vi "1BS3HD_Convert_HD_v00.vi"(8 "Extras Homodyne":T1, 11 "PII Control":T2={"P Gain"=0, "P Bit Shift"=1, "I Bit Shift"=0, "I Gain"=1, "Lock Threshold"=20, "Lock"=FALSE, "Hold"=FALSE, "Scan Frequency"=65509, "Scan Bit Shift"=20, "Gains +/- "=FALSE, "Pre- Offset x"=-5.0, "Pre-Offset p"=8.0, "Gain Error x"=-5, "Lock Angle"=0.0, "Gain Error p\n\n"=-4} {"Lock Angle" min=-90.0 max=90.0 scale=-90.0..90.0 scale format="%#_2g"; "Pre-Offset p" scale=-0.01..0.01 scale format="%#_5f"; "Pre- Offset x" scale=-0.01..0.01 scale format="%#_5f"; "Scan Frequency" scale=1.0..30.0; "I Gain" scale=0.0..50.0; "P Gain" scale=0.0..50.0}) -> (3 "PII+Error":T11)   [LabVIEW 2013]
uses:
  Strict Type Defs/PII individual.ctl
  Strict Type Defs/Errors Converted Graph HD.ctl
  Strict Type Defs/PII and Error Graph HD.ctl
  Strict Type Defs/1BS3HD Control GUI HD.ctl
  Strict Type Defs/PII Gains.ctl
  Strict Type Defs/I16 white control.ctl
  Strict Type Defs/Thresh slider.ctl
  Strict Type Defs/Lock or Hold.ctl
  Strict Type Defs/Scan Freq Slider.ctl
  Strict Type Defs/Gains negative horizontal.ctl
  Strict Type Defs/Slider and display.ctl
  Strict Type Defs/theta 1SDI.ctl
  Strict Type Defs/Extras PII 1SDI HD.ctl
panel:
  in  "PII+Error type def":T11
  in  "Error individual":T12
  in  "PII In typdef":T13
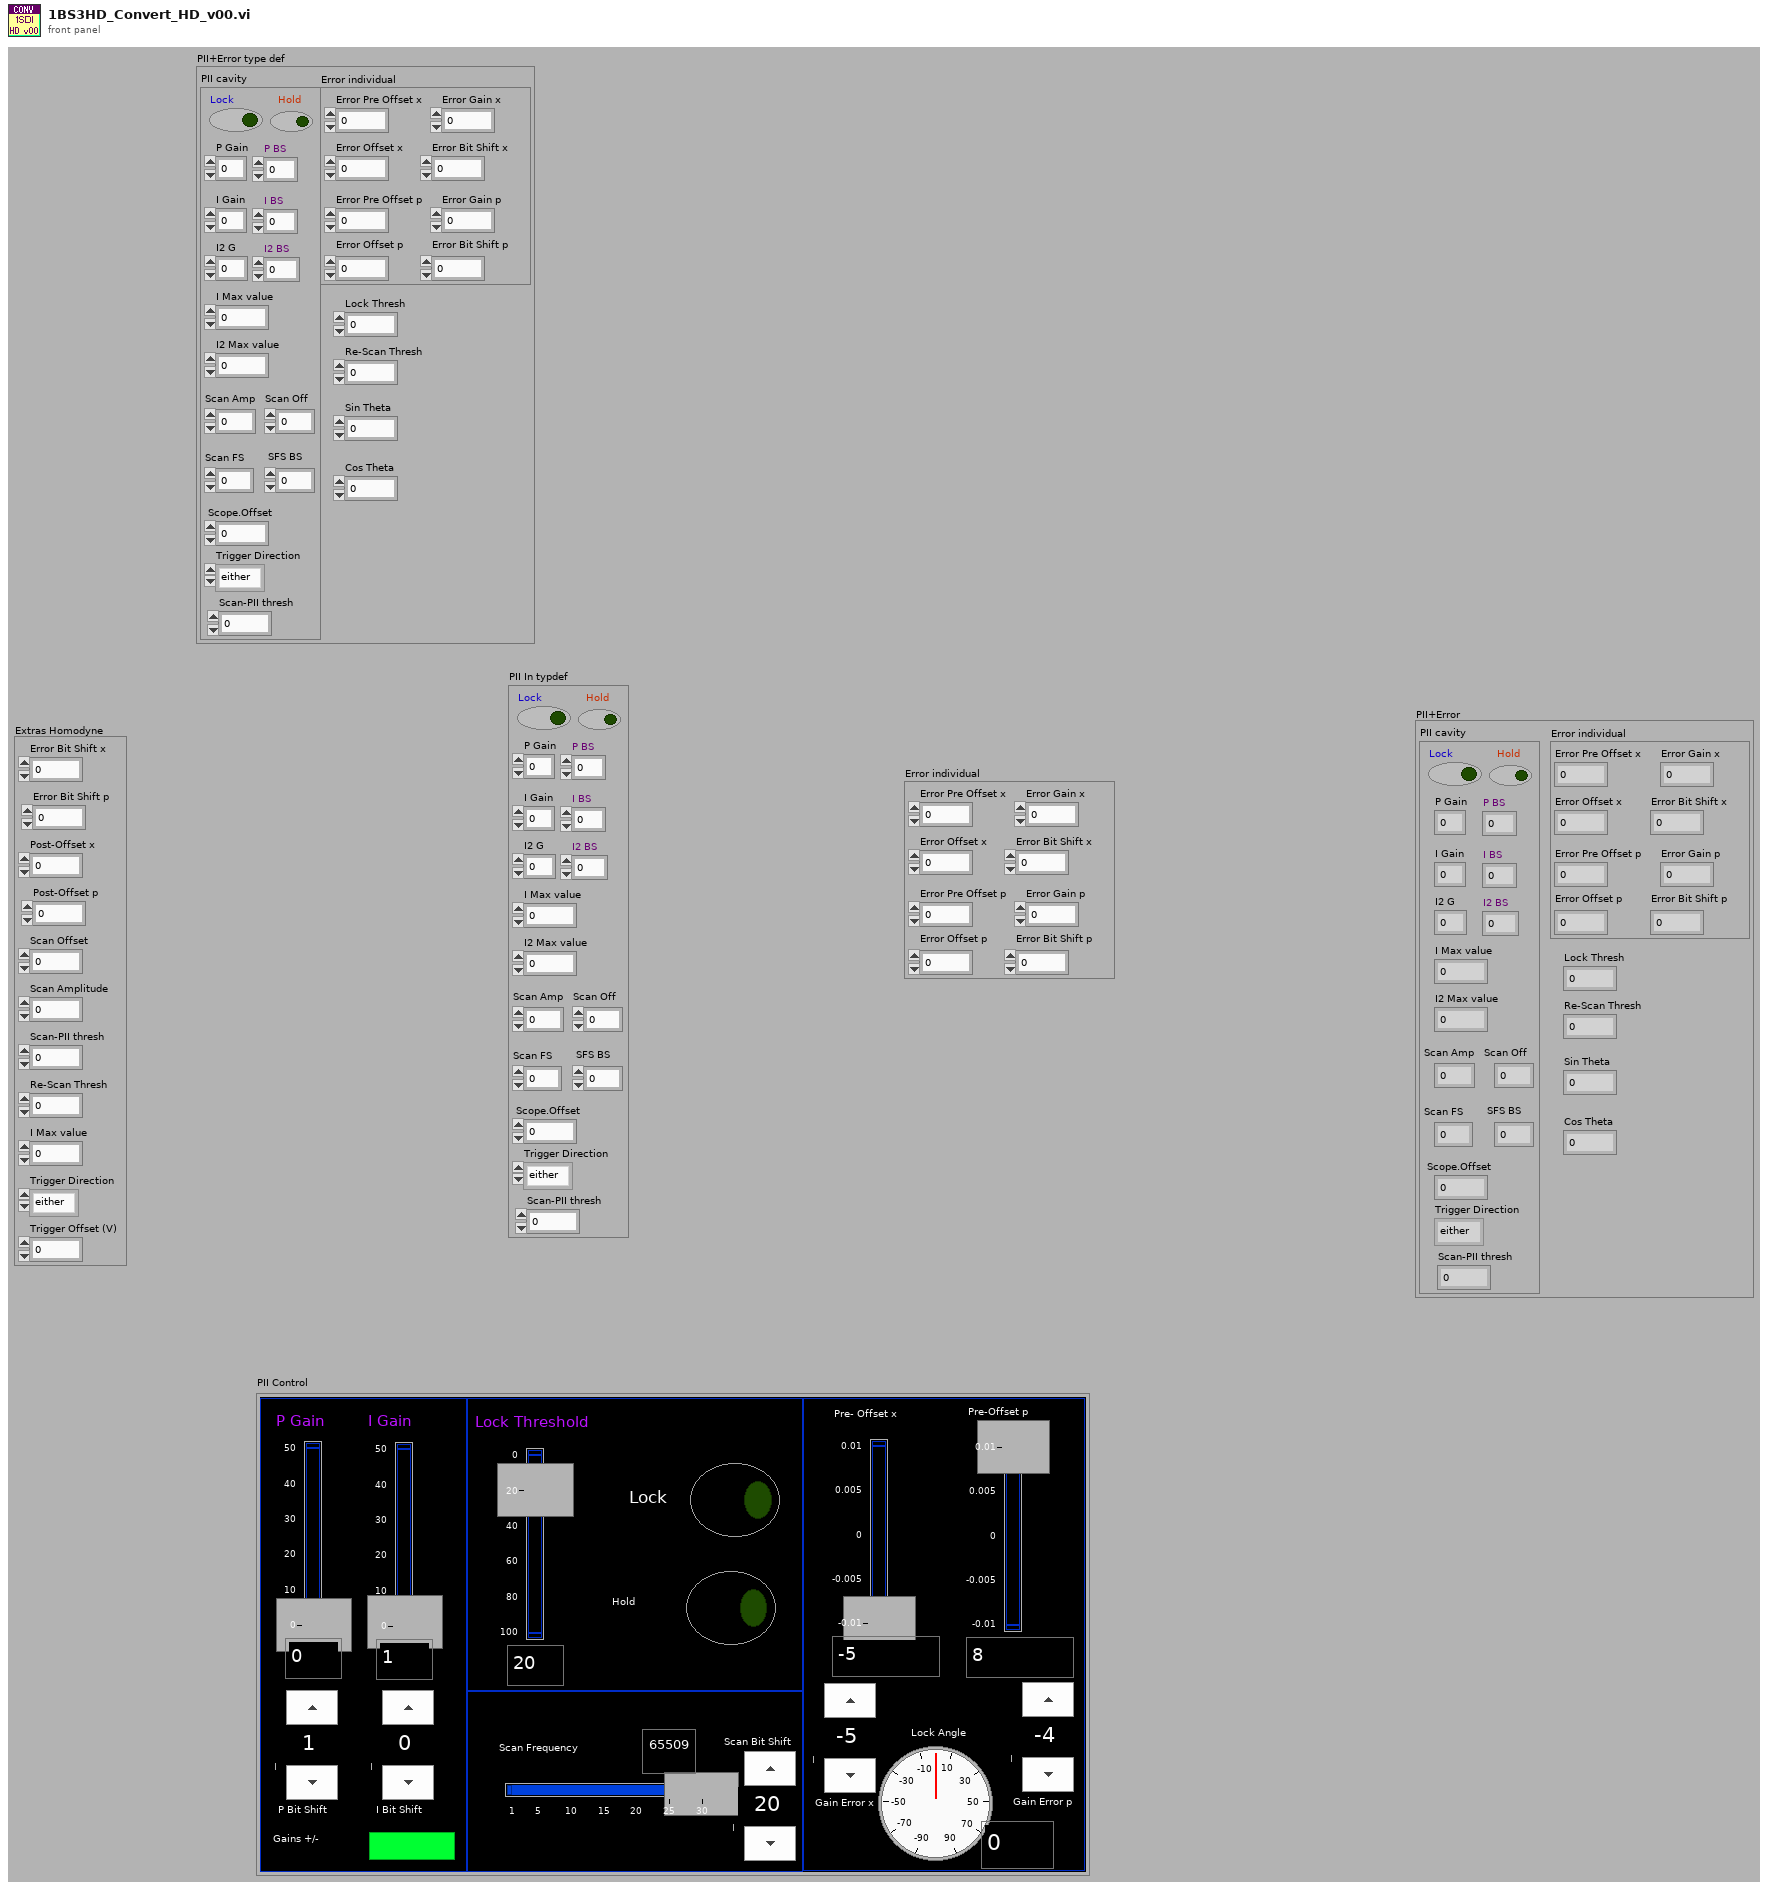
[diagram p1: front panel]
types:
  T1 = typedef "Extras PII 1SDI HD.ctl" = cluster{"Error Bit Shift p":i16, "Scan Offset":dbl, "Scan Amplitude":dbl, "Scan-PII thresh":i16, "Re-Scan Thresh":i16, "I Max value":i32, "Trigger Direction":enum8{"either", "minus-plus", "plus-minus"}, "Trigger Offset (V)":dbl, "Error Bit Shift x":i16, "Post-Offset p":dbl, "Post-Offset x":dbl}
  T2 = typedef "1BS3HD Control GUI HD.ctl" = cluster{"P Gain":T3, "P Bit Shift":T4, "I Bit Shift":T4, "I Gain":T3, "Lock Threshold":T5, "Lock":T6, "Hold":T6, "Scan Frequency":T7, "Scan Bit Shift":T4, "Gains +/- ":T8, "Pre- Offset x":T9, "Pre-Offset p":T9, "Gain Error x":T4, "Lock Angle":T10, "Gain Error p\n\n":T4}
  T3 = typedef "PII Gains.ctl" = i32
  T4 = typedef "I16 white control.ctl" = i16
  T5 = typedef "Thresh slider.ctl" = i16
  T6 = typedef "Lock or Hold.ctl" = bool
  T7 = typedef "Scan Freq Slider.ctl" = u16
  T8 = typedef "Gains negative horizontal.ctl" = bool
  T9 = typedef "Slider and display.ctl" = dbl
  T10 = typedef "theta 1SDI.ctl" = dbl
  T11 = typedef "PII and Error Graph HD.ctl" = cluster{"Error individual":T12, "PII cavity":T13, "Lock Thresh":i16, "Re-Scan Thresh":i16, "Sin Theta":i32, "Cos Theta":i32}
  T12 = typedef "Errors Converted Graph HD.ctl" = cluster{"Error Pre Offset x":i16, "Error Offset x":i16, "Error Gain x":i16, "Error Bit Shift x":i16, "Error Pre Offset p":i16, "Error Offset p":i16, "Error Gain p":i16, "Error Bit Shift p":i16}
  T13 = typedef "PII individual.ctl" = cluster{"Lock":bool, "Hold":bool, "P Gain":i32, "P BS":i16, "I Gain":i32, "I BS":i16, "I2 G":i32, "I2 BS":i16, "Scan Amp":i16, "Scan Off":i16, "Scan FS":u16, "SFS BS":i16, "I Max value":i32, "I2 Max value":i32, "Scope.Offset":i16, "Trigger Direction":enum8{"either", "minus-plus", "plus-minus"}, "Scan-PII thresh":i16}
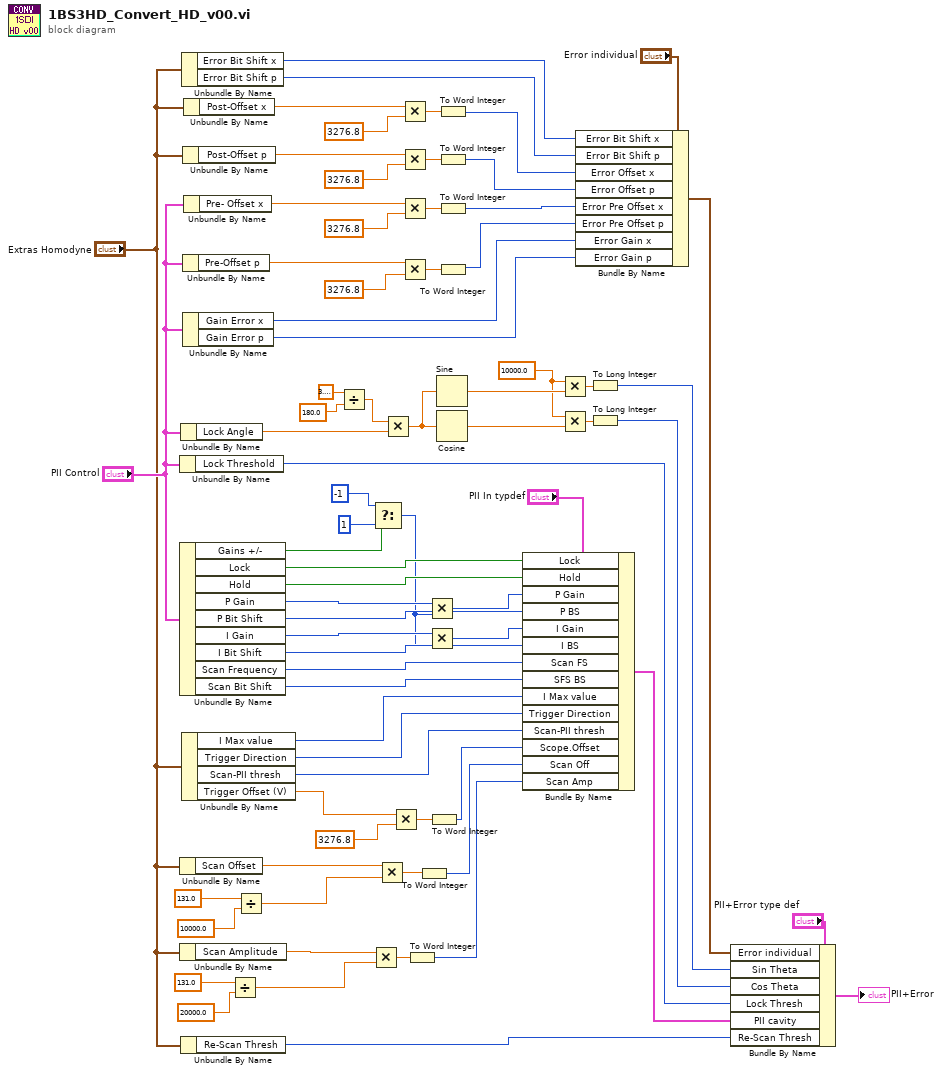
[diagram p0: block diagram]
diagram:
  w17 = T10 10000.0 ("x")
  n1 = Unbundle By Name("PII Control") -> ("Lock Threshold"=w38:T5)
  n2 = Unbundle By Name("PII Control") -> ("Gains +/-"=w56:T8, "Lock"=w60:T6, "Hold"=w59:T6, "P Gain"=w55:T3, "P Bit Shift"=w58:T4, "I Gain"=w51:T3, "I Bit Shift"=w57:T4, "Scan Frequency"=w48:T7, "Scan Bit Shift"=w47:T4)
  n3 = Unbundle By Name("Extras Homodyne") -> ("Scan Offset"=w39:dbl)
  n4 = Unbundle By Name("Extras Homodyne") -> ("Scan Amplitude"=w70:dbl)
  n5 = Unbundle By Name("PII Control") -> ("Lock Angle"=w21:T10)
  n6 = Unbundle By Name("Extras Homodyne") -> ("Re-Scan Thresh"=w28:i16)
  n7 = Unbundle By Name("Extras Homodyne") -> ("Error Bit Shift x"=w11:i16, "Error Bit Shift p"=w12:i16)
  n8 = Unbundle By Name("Extras Homodyne") -> ("I Max value"=w36:i32, "Trigger Direction"=w35:enum8{"either", "minus-plus", "plus-minus"}, "Scan-PII thresh"=w34:i16, "Trigger Offset (V)"=w30:dbl)
  n9 = Unbundle By Name("Extras Homodyne") -> ("Post-Offset p"=w6:dbl)
  n10 = Unbundle By Name("PII Control") -> ("Pre-Offset p"=w71:T9)
  n11 = Unbundle By Name("PII Control") -> ("Gain Error x"=w41:T4, "Gain Error p"=w1:T4)
  n12 = Unbundle By Name("Extras Homodyne") -> ("Post-Offset x"=w8:dbl)
  n13 = Unbundle By Name("PII Control") -> ("Pre- Offset x"=w13:T9)
  n14 = Divide(x=131.0, y=20000.0) -> (x/y=w65:dbl)
  n15 = Divide(x=131.0, y=10000.0) -> (x/y=w62:dbl)
  n16 = Divide(x=3.141592653589793, y=180.0) -> (x/y=w22:dbl)
  n17 = Multiply(x=w70, y=w65) -> (x*y=w68:dbl)
  n18 = Select(t=T3 -1 ("y"), s=w56, f=T3 1) -> (s? t:f=w49:T3)
  n19 = Multiply(x=w39, y=w62) -> (x*y=w69:dbl)
  n20 = Multiply(x=w22, y=w21) -> (x*y=w25:T10)
  n21 = Multiply(x=w30, y=3276.8) -> (x*y=w32:dbl)
  n22 = Multiply(x=w8, y=3276.8) -> (x*y=w10:dbl)
  n23 = Multiply(x=w6, y=3276.8) -> (x*y=w4:dbl)
  n24 = Multiply(x=w13, y=3276.8) -> (x*y=w74:T9)
  n25 = Multiply(x=w71, y=3276.8) -> (x*y=w73:T9)
  n26 = To Word Integer(number=w68) -> (16bit integer=w37:i16)
  n27 = To Word Integer(number=w69) -> (16bit integer=w33:i16)
  n28 = Multiply(x=w55, y=w49) -> (x*y=w52:T3)
  n29 = Multiply(x=w51, y=w49) -> (x*y=w50:T3)
  n30 = To Word Integer(number=w32) -> (16bit integer=w29:i16)
  n31 = Sine(x=w25) -> (sin(x)=w20:T10)
  n32 = Cosine(x=w25) -> (cos(x)=w18:T10)
  n33 = To Word Integer(number=w10) -> (16bit integer=w7:i16)
  n34 = To Word Integer(number=w4) -> (16bit integer=w2:i16)
  n35 = To Word Integer(number=w74) -> (16bit integer=w45:i16)
  n36 = To Word Integer(number=w73) -> (16bit integer=w44:i16)
  n37 = Bundle By Name(cluster="PII In typdef", "Lock"=w60, "Hold"=w59, "P Gain"=w52, "P BS"=w58, "I Gain"=w50, "I BS"=w57, "Scan FS"=w48, "SFS BS"=w47, "I Max value"=w36, "Trigger Direction"=w35, "Scan-PII thresh"=w34, "Scope.Offset"=w29, "Scan Off"=w33, "Scan Amp"=w37) -> (w42:T13)
  n38 = Multiply(x=w17, y=w20) -> (x*y=w26:T10)
  n39 = Multiply(x=w17, y=w18) -> (x*y=w19:T10)
  n40 = Bundle By Name(cluster="Error individual", "Error Bit Shift x"=w11, "Error Bit Shift p"=w12, "Error Offset x"=w7, "Error Offset p"=w2, "Error Pre Offset x"=w45, "Error Pre Offset p"=w44, "Error Gain x"=w41, "Error Gain p"=w1) -> (w27:T12)
  n41 = To Long Integer(number=w26) -> (32bit integer=w15:i32)
  n42 = To Long Integer(number=w19) -> (32bit integer=w16:i32)
  n43 = Bundle By Name(cluster="PII+Error type def", "Error individual"=w27, "Sin Theta"=w15, "Cos Theta"=w16, "Lock Thresh"=w38, "PII cavity"=w42, "Re-Scan Thresh"=w28) -> (→"PII+Error":T11)
